vi "Teste.vi"() -> ()   [LabVIEW 2017]
panel:
  out "Posição desejada (juntas)":dbl[](array[numeric])
  in  "Posição desejada (roll, pitch, yaw)":dbl[](array[numeric])
  in  "Posição atual (juntas)":dbl[](array[numeric])
  in  "Posição desejada (x,y,z)":dbl[](array[numeric])
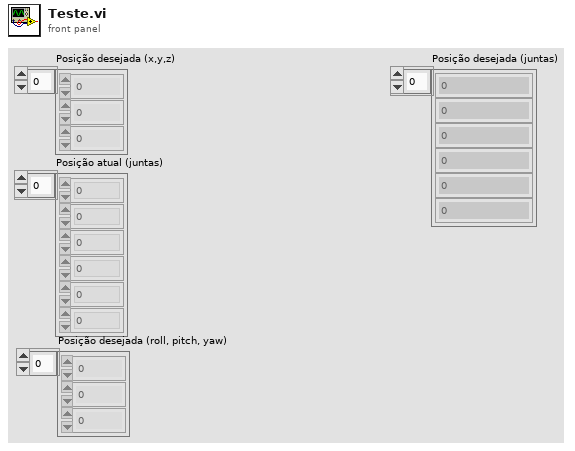
[diagram p1: front panel]
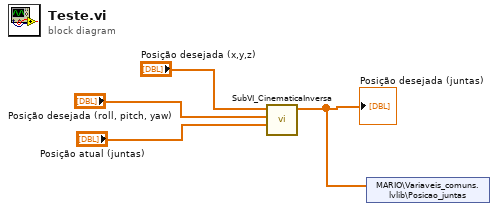
[diagram p0: block diagram]
diagram:
  n1 = call "SubVI_CinematicaInversa.vi"("Posição desejada (x,y,z)"="Posição desejada (x,y,z)", "Posição desejada (roll, pitch, yaw)"="Posição desejada (roll, pitch, yaw)", "Posição atual (juntas)"="Posição atual (juntas)") -> ("Posição desejada (juntas)"=w1:dbl[])  [unwired: 6 in, 1 out]
  "Posição desejada (juntas)" <- w1
  n2 = shared-variable "MARIO\\Variaveis_comuns.lvlib\\Posicao_juntas"(w1) -> ()  [unwired: 1 in, 1 out]
